vi "find device.vi"(11 "search string":string="USRP") -> (3 "resource name":T1[](array[typedef]))   [LabVIEW 2022 SP3]
uses:
  <vilib>/userDefined/High Color/nirio_resource_hc.ctl
  <vilib>/nisyscfg/Filter Mode.ctl
  <vilib>/nisyscfg/nisyscfg.lvlib
  <resource>/objmgr/niflexrioatomicsae.rc
panel:
  in  "Target (localhost)":refnum<k21>="localhost"
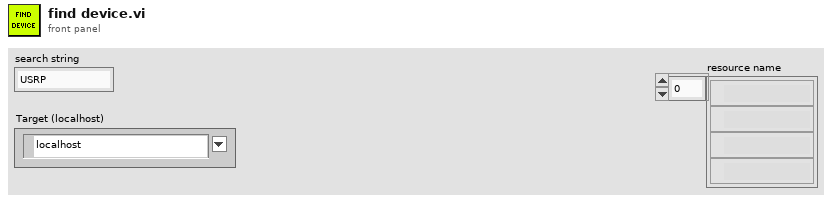
[diagram p1: front panel]
types:
  T1 = typedef "nirio_resource_hc.ctl" = tag
  T2 = typedef "nisyscfg.lvlib/Filter Mode.ctl" = i32
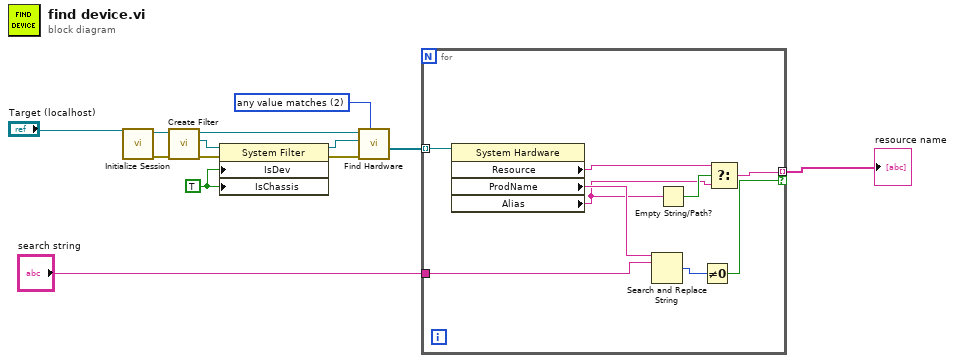
[diagram p0: block diagram]
diagram:
  w3 = T2 2 items=["all values match"=1, "any value matches"=2, "values do not match"=3, "all properties exist"=4] ("Filter Mode (all values match)")
  w5 = TRUE ("Is Chassis")
  n1 = call <vilib>:"Initialize Session.vi"("Target (localhost)"="Target (localhost)") -> ("error out"=w8:errorcluster, "Session out"=w11:refnum<k21>)  [unwired: 9 in]
  n2 = call <vilib>:"Create Filter.vi"("error in (no error)"=w8, "Session in"=w11) -> ("error out"=w13:errorcluster, "Filter out"=w12:refnum<k20>, "Session out"=w10:refnum<k21>)  [unwired: 7 in]
  n3 = property class="System Filter"(reference=w12, error in=w13, "IsDev"=w5, "IsChassis"=w5) -> (reference out=w7:refnum<k20>, error out=w9:errorcluster)
  n4 = call <vilib>:"Find Hardware.vi"("Filter Mode (all values match)"=w3, "error in (no error)"=w9, "Filter in"=w7, "Session in"=w10) -> ("Resources out"=w4:refnum<k20>[])  [unwired: 7 out]
  n5 = for {
    tunnel: w4 -> [w22] mode=indexing
    tunnel: [w14] -> w1 mode=indexing if=w19
    tunnel: "search string" -> [w18]
    n6 = property class="System Hardware"(reference=w22) -> ("Resource"=w16:string, "ProdName"=w21:string, "Alias"=w15:string)  [unwired: 1 in, 2 out]
    n7 = Search and Replace String(input string=w21, search string=w18) -> (number of replacements=w20:i32)  [unwired: 6 in, 3 out]
    n8 = Empty String/Path?(string/path=w15) -> (empty?=w17:bool)
    n9 = Not Equal To 0?(x=w20) -> (x != 0?=w19:bool)
    n10 = Select(t=w16, s=w17, f=w15) -> (s? t:f=w14:string)
  }
  "resource name" <- w1
